vi "Ctor.vi"(8 "error in (no error)":errorcluster, 11 "ElementEditorPanel in":refnum<class "ElementEditorPanel.lvclass">) -> (0 "error out":errorcluster, 3 "ElementEditorPanel out":refnum<class "ElementEditorPanel.lvclass">)   [LabVIEW 2020, in "VolatusGUIEditorCore.lvlib" / "ElementEditorPanel.lvclass"]
uses:
  ElementEditorPanel.lvclass
  lv-oopanel/OOPanel/Panel/Panel.lvclass
  ElementEditorPanel.lvclass/ElementEditorPanel.ctl
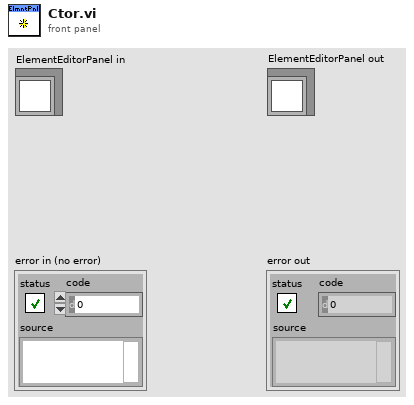
[diagram p1: front panel]
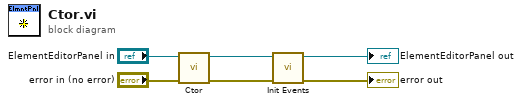
[diagram p0: block diagram]
diagram:
  n1 = call-parent "Ctor.vi"("error in (no error)"="error in (no error)", "Panel in"="ElementEditorPanel in") -> ("error out"=w5:errorcluster, "Panel out"=w2:refnum<class "ElementEditorPanel.lvclass">)  [unwired: 8 in]
  n2 = call "Init Events.vi"("error in (no error)"=w5, "ElementEditorPanel in"=w2) -> ("error out"=→"error out":errorcluster, "ElementEditorPanel out"=→"ElementEditorPanel out":refnum<class "ElementEditorPanel.lvclass">)  [unwired: 8 in]
